vi "Update GUI - Reset Waveform Chart.vi"(8 "error in (no error)":errorcluster, 10 "GUI Item Name":string, 11 "uService Template in":refnum<class "Father of all uServices.lvclass">) -> (0 "error out":errorcluster, 3 "uService Template out":refnum<class "Father of all uServices.lvclass">)   [LabVIEW 2026, in "TALOS.lvlib" / "Father of all uServices.lvlib" / "Father of all uServices.lvclass"]
doc: "This VI reset the Waveform Chart to its default data."
uses:
  Father of all uServices.lvclass
  Waveform Chart Class Reference Strict - single plot.ctl
  Ancestor/Ancestor/Ancestor.lvclass/Ancestor.ctl
  Support VIs/Generate Error.vi
  FGV/Error Memory/Get Error Description.vi
  Support VIs/Get PC name.vi
  Ancestor/Ancestor/Read ID.vi
  Support VIs/Get Class Name.vi
  <vilib>/Utility/error.llb/Clear Errors.vi
  FGV/Error Memory/Error Memory Core.vi
  <vilib>/AdvancedString/Delimited String to 1D String Array.vi
  <vilib>/AdvancedString/Delimited String to 1D String Array (string).vi
  Support VIs/Circus Root Path.vi
  FGV/Error Memory/Error Crt Lvl checker.vi
  FGV/Error Memory/Error Memory Core.vi/40c8088d-b597-4017-91af-faa98e00292e.vi
  FGV/Error Memory/Error Memory Core.vi/d4a3ab98-063c-4e44-b43d-fbdcfe6c2be2.vi
  Support VIs/Global Memory.vi
  <vilib>/Utility/LVClass/Get LV Class Name.vi
  Support VIs/Is in Packed Library.vi
  Support VIs/TALOS Root path.vi
  Support VIs/Read CSV worksheet.vi
  Support VIs/Global Constants.vi
  <vilib>/Utility/error.llb/General Error Handler.vi
  Support VIs/Error Log.vi
  Ancestor/Ancestor/Ancestor.lvclass
  <vilib>/Comparison/Equal/Equal Functor/Equal Functor.lvclass
  TALOS.lvlib
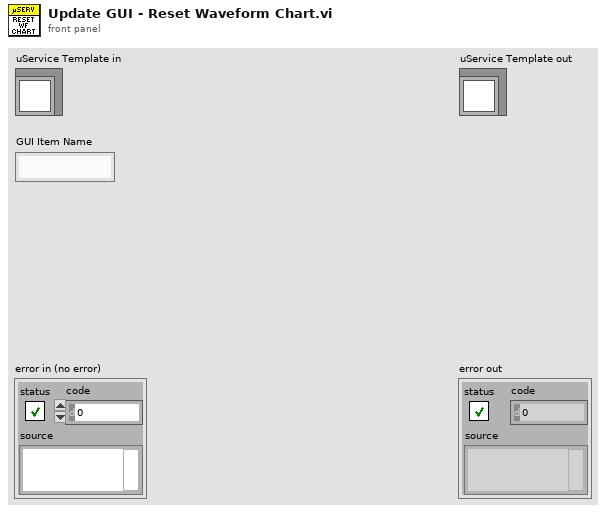
[diagram p1: front panel]
types:
  T1 = typedef "TALOS.lvlib/Father of all uServices.lvlib/Father of all uServices.lvclass/Waveform Chart Class Reference Strict - single plot.ctl" = refnum<vi>
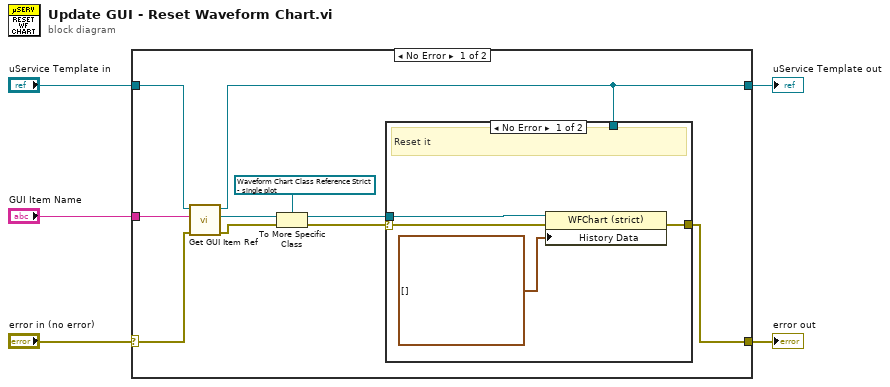
[diagram p0: block diagram]
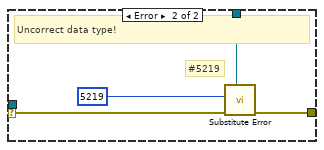
[diagram p2: hidden frame]
diagram:
  n1 = case shown="No Error" "error in (no error)" {
    selector: "error in (no error)" -> [w13 w25]
    tunnel: [w7 w25] -> w4
    tunnel: [w8 w24] -> w2
    tunnel: "uService Template in" -> [w14 w24]
    tunnel: "GUI Item Name" -> [w15 _]
    frame No Error {
      n2 = call "Get GUI Item Ref.vi"("error in (no error)"=w13, "FP Item Name"=w15, "uService Template in"=w14) -> ("error out"=w11:errorcluster, "Ctl Refnum"=w12:refnum<vi>, "uService Template out"=w8:refnum<class "Father of all uServices.lvclass">)  [unwired: 6 in]
      n3 = To More Specific Class(target class=T1 refnum, reference=w12, error in=w11) -> (specific class reference=w10:T1, error out=w9:errorcluster)
      n4 = case shown="No Error" w9 {
        selector: w9 -> [w18 w23]
        tunnel: w10 -> [w19 _]
        tunnel: w8 -> [_ w22]
        tunnel: [w17 w20] -> w7
        frame No Error {
          # "Reset it"
          n5 = property class="WFChart (strict)"(reference=w19, error in=w18, "History Data"=waveform(dbl)[] []) -> (error out=w17:errorcluster)  [unwired: 1 out]
        }
        frame Error {
          # "#5219"
          # "Uncorrect data type!"
          n6 = call "Substitute Error.vi"("LabVIEW Object"=w22, "error in (no error)"=w23, "Error Code"=5219) -> ("error out"=w20:errorcluster)  [unwired: 8 in]
        }
      }
    }
    frame Error {
    }
  }
  "error out" <- w4
  "uService Template out" <- w2
